vi "XY Graph TipStrip Event Registration.vi"(8 "error in (no error)":errorcluster, 11 "XY Graph Refnum":T1) -> (0 "error out":errorcluster, 2 "Event Registration Refnum":refnum<event-registration>, 3 "XY Graph Refnum":T1)   [LabVIEW 2021, in "XY Graph Add-Ons.lvlib"]
uses:
  XY Graph/XY Graph Add-Ons.lvlib
  XY Graph/XY Graph Refnum.ctl
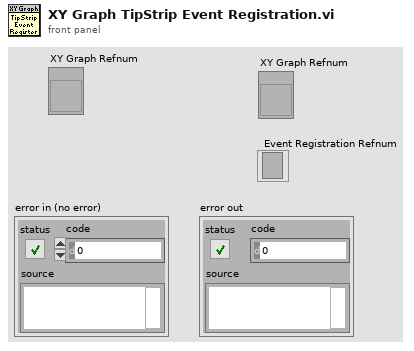
[diagram p1: front panel]
types:
  T1 = typedef "XY Graph Add-Ons.lvlib/XY Graph Refnum.ctl" = refnum<vi>
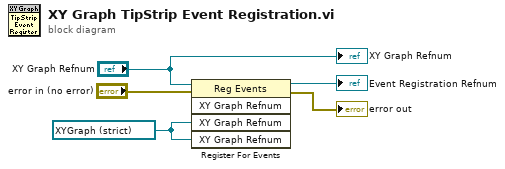
[diagram p0: block diagram]
diagram:
  w4 = refnum<vi> refnum ("XY Graph Refnum")
  n1 = register-events(error in="error in (no error)", "XY Graph Refnum", w4, w4) -> (reference out=→"Event Registration Refnum":refnum<event-registration>, error out=→"error out":errorcluster)  [unwired: 1 in]
  "XY Graph Refnum" <- "XY Graph Refnum"
